vi "DAQChannelReadWaveform.vi"(5 "DAQ Channel Name Input":tag) -> (1 "Waveform Cluster":cluster{"t0":timestamp, "dt":dbl, "Y":dbl[]} {"Y" format="%0.2f"; "dt" format="%0.2f"; "t0" format="%<%X\n%x>T"}, 2 "DAQ Channel Name Output":tag)   [LabVIEW 2011]
uses:
  <vilib>/Daq/1easyio.llb/AI Acquire Waveform (waveform).vi
panel:
  out "waveform":waveform(dbl)(graph)
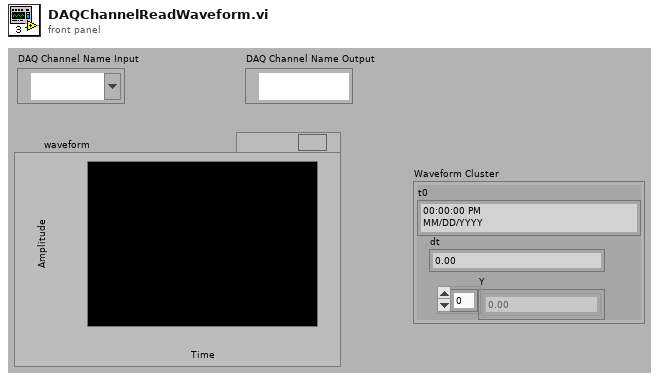
[diagram p1: front panel]
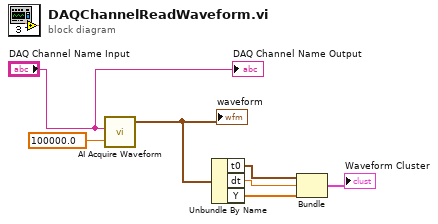
[diagram p0: block diagram]
diagram:
  n1 = call-poly <vilib>:"AI Acquire Waveform.vi"("sample rate (1000 samples/sec)"=sgl 100000.0, "channel (0)"="DAQ Channel Name Input") -> ("waveform"=w5:waveform(dbl))  [unwired: 2 in, 4 out]
  "waveform" <- w5
  n2 = Unbundle By Name(w5) -> ("t0"=w4:timestamp, "dt"=w3:dbl, "Y"=w2:dbl[])
  n3 = Bundle("t0"=w4, "dt"=w3, "Y"=w2) -> (→"Waveform Cluster":cluster{"t0":timestamp, "dt":dbl, "Y":dbl[]})  [unwired: 1 out]
  "DAQ Channel Name Output" <- "DAQ Channel Name Input"
